vi "Dequeue Published Result by Type.vi"(8 "error in (no error)":errorcluster, 9 "timeout in ms":i32, 10 "Result Type":T1, 11 "Mock Result Observer In":refnum<class "Mock Result Observer.lvclass">) -> (0 "error out":errorcluster, 1 "timed out?":bool, 2 "Result":T2, 3 "Mock Result Observer Out":refnum<class "Mock Result Observer.lvclass">)   [LabVIEW 2020, in "Mock Result Observer.lvclass"]
uses:
  Mock Result Observer.lvclass
  Result/Result.ctl
  Result/Status.ctl
  Result/Type.ctl
  Mock Result Observer.lvclass/Mock Result Observer.ctl
  Result/Result.lvlib
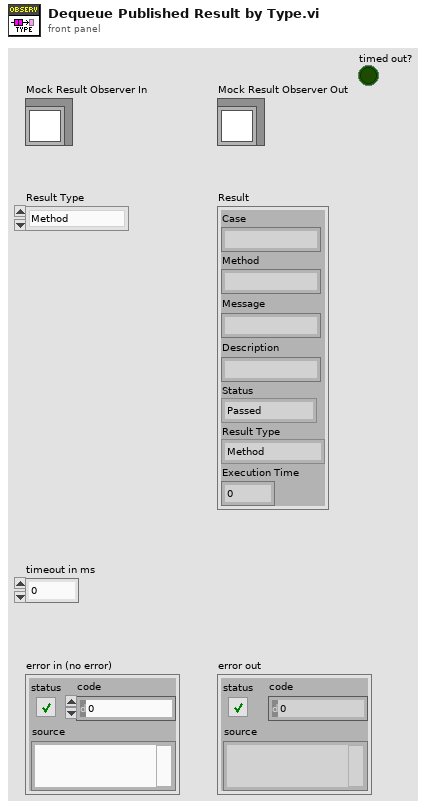
[diagram p1: front panel]
types:
  T1 = typedef "Result.lvlib/Type.ctl" = enum16{"Method", "Case", "Suite", "Pass", "Fail", "Skip", "Pass if", "Fail if", "Pass if Error", "Fail if Error", "Pass if Equal", "Fail if Equal"}
  T2 = typedef "Result.lvlib/Result.ctl" = cluster{"Case":string, "Method":string, "Message":string, "Description":string, "Status":T3, "Result Type":T1, "Execution Time":dbl}
  T3 = typedef "Result.lvlib/Status.ctl" = enum16{"Passed", "Failed", "Error", "Skipped", "Setup Error", "Broken", "Teardown Error"}
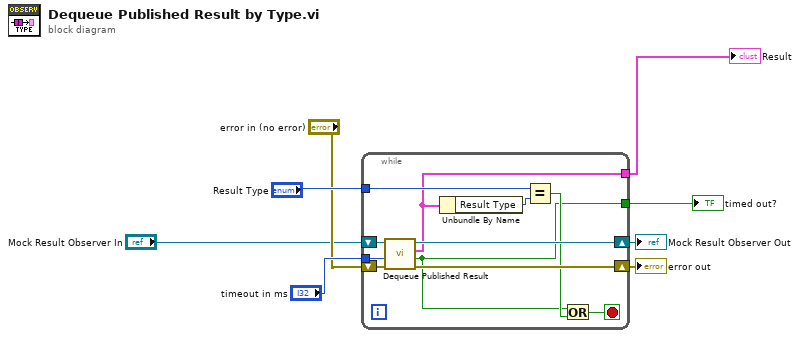
[diagram p0: block diagram]
diagram:
  n1 = while {
    tunnel: "timeout in ms" -> [w15]
    shift-right: [w19] -> w2
    shift-left: "Mock Result Observer In" -> [w17]
    shift-right: [w18] -> w3
    shift-left: "error in (no error)" -> [w16]
    tunnel: "Result Type" -> [w14]
    tunnel: [w10] -> w8
    tunnel: [w9] -> w1
    stop <- w12 stop-if-true
    n2 = call "Dequeue Published Result.vi"("error in (no error)"=w16, "timeout in ms (-1)"=w15, "Mock Result Observer In"=w17) -> ("error out"=w18:errorcluster, "timed out?"=w9:bool, "Result"=w10:T2, "Mock Result Observer Out"=w19:refnum<class "Mock Result Observer.lvclass">)  [unwired: 5 in]
    n3 = Unbundle By Name(w10) -> ("Result Type"=w13:T1)
    n4 = Equal?(x=w14, y=w13) -> (x = y?=w11:bool)
    n5 = Or(x=w9, y=w11) -> (x .or. y?=w12:bool)
  }
  "Result" <- w8
  "error out" <- w3
  "Mock Result Observer Out" <- w2
  "timed out?" <- w1
